vi "Add Child to Document.vi"(8 "error in (no error)":errorcluster, 9 "Tag Name":string, 11 "DOM document":refnum<k20>) -> (0 "error out":errorcluster, 2 "Child Element":refnum<k20>, 3 "DOM document out":refnum<k20>)   [LabVIEW 2013]
uses:
  <resource>/objmgr/DOMUserDefRef.rc
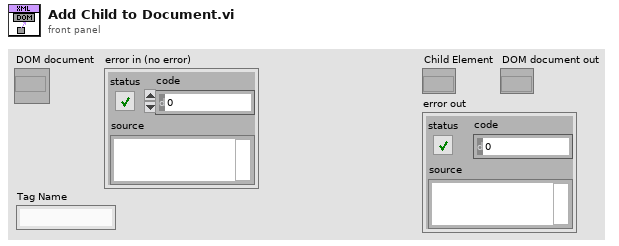
[diagram p1: front panel]
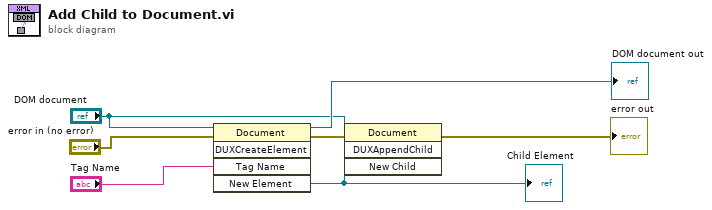
[diagram p0: block diagram]
diagram:
  n1 = invoke class="Document" method="DUXCreateElement"(reference="DOM document", error in="error in (no error)", "Tag Name"="Tag Name") -> (reference out=→"DOM document out":refnum<k20>, error out=w5:errorcluster, "New Element"=w4:refnum<k20>)  [unwired: 2 in, 2 out]
  "Child Element" <- w4
  n2 = invoke class="Document" method="DUXAppendChild"(reference="DOM document", error in=w5, "New Child"=w4) -> (error out=→"error out":errorcluster)  [unwired: 1 in, 3 out]
